vi "operate.vi"(8 "error in (no error)":errorcluster, 11 "reference in":refnum<class "GUI Controller.lvclass">) -> (0 "error out":errorcluster, 3 "reference out":refnum<class "GUI Controller.lvclass">)   [LabVIEW 2015, in "GUI Controller.lvclass"]
uses:
  GUI Controller.lvclass
  products.ctl
  inventory.ctl
  APP/excelFile_class/fileType.ctl
  followUp.ctl
  partsTracking.ctl
  state.ctl
  Project Panels_class/Project Panels.lvclass
  SYS/Items Controller_llb/Items Controller.lvclass
  APP/excelFile_class/excelFile.lvclass
  SYS/Notification Controller_class/Notification Controller.lvclass
  SYS/PartsTracking Controller_class/PartsTracking Controller.lvclass
  SYS/File Controller_llb/File Controller.lvclass
panel:
  out "Title":string
  in  "Parts Tracking":T1
  in  "Follow up":T2
  in  "fileType":T3
  in  "Settings Button":bool
  in  "Inventory":T4
  in  "Products":T5
  out "StatusBar":string
  in  "Stop Button":bool
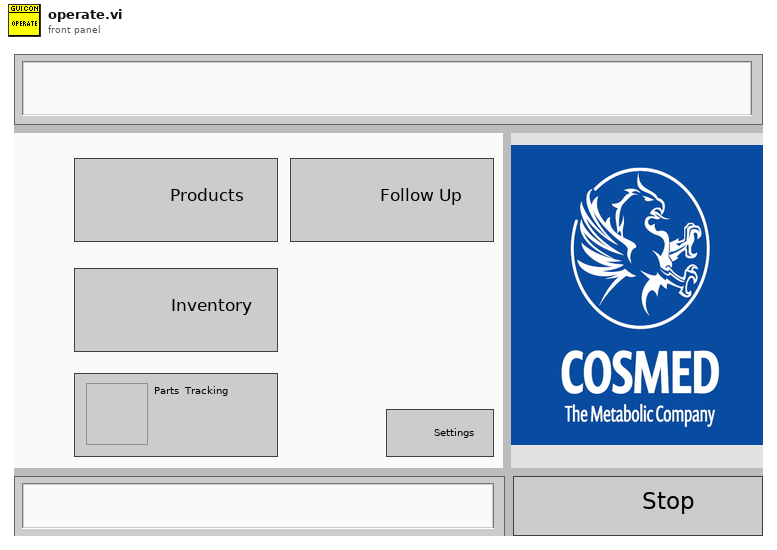
[diagram p1: front panel]
types:
  T1 = typedef "GUI Controller.lvclass/partsTracking.ctl" = bool
  T2 = typedef "GUI Controller.lvclass/followUp.ctl" = bool
  T3 = typedef "excelFile.lvclass/fileType.ctl" = enum16{"devices", "items", "partsTracking"}
  T4 = typedef "GUI Controller.lvclass/inventory.ctl" = bool
  T5 = typedef "GUI Controller.lvclass/products.ctl" = bool
  T6 = typedef "GUI Controller.lvclass/state.ctl" = enum16{"initiate", "checkNotificationItems", "checkNotificationTracking", "operate", "updateFromFile", "stop"}
  T7 = enum32{"Invalid", "Standard", "Closed", "Hidden", "Minimized", "Maximized"}
  T8 = typedef "GUI Controller.lvclass/ObjectAttributesRef.ctl" = refnum<data-value>
  T9 = typedef "GUI Controller.lvclass/ObjectAttributes.ctl" = cluster{"MyAttribute":dbl, "state":T6, "project_panels_ref":refnum<class "Project Panels.lvclass">, "items_controller_ref":refnum<class "Items Controller.lvclass">, "notification_controller_ref":refnum<class "Notification Controller.lvclass">, "partstracking_controller_ref":refnum<class "PartsTracking Controller.lvclass">, "file_controller_ref":refnum<class "File Controller.lvclass">}
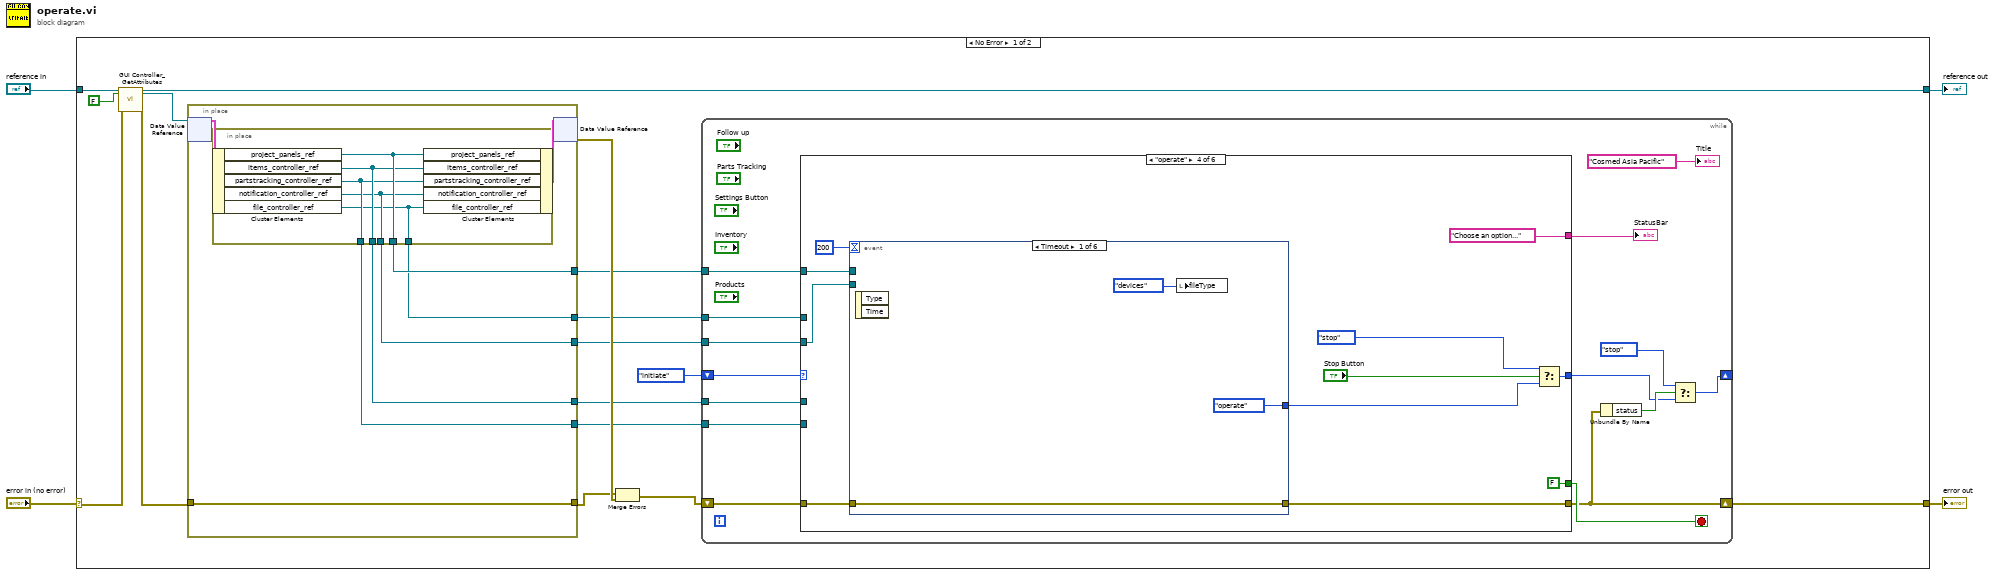
[diagram p0: block diagram]
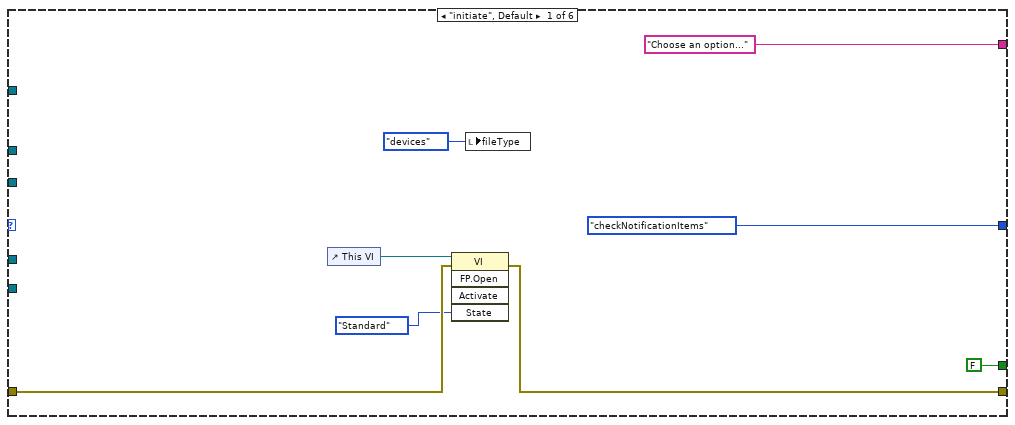
[diagram p2: hidden frame]
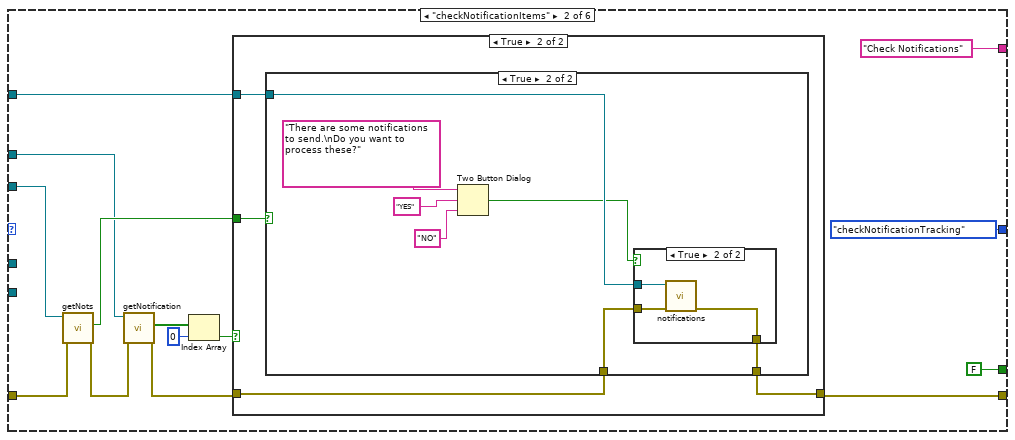
[diagram p3: hidden frame]
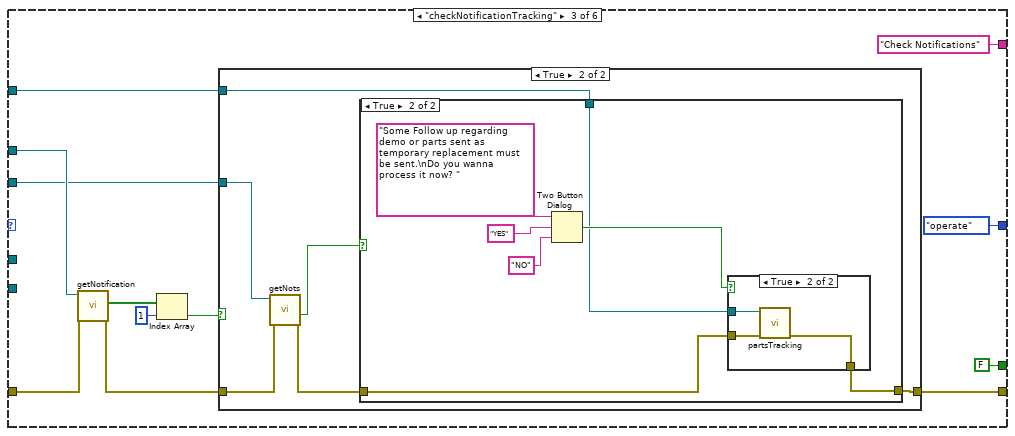
[diagram p7: hidden frame]
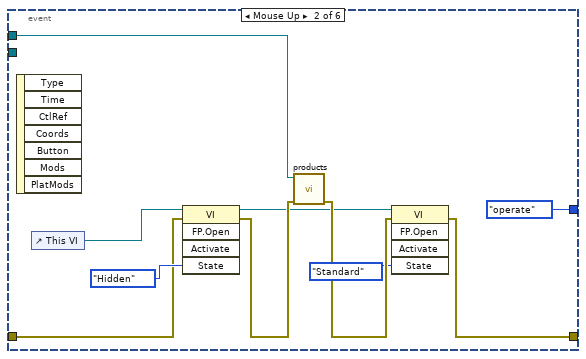
[diagram p11: hidden frame]
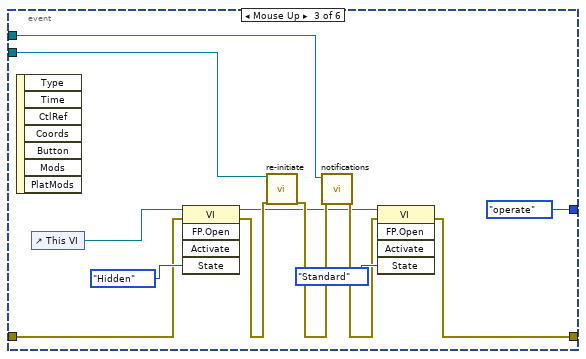
[diagram p12: hidden frame]
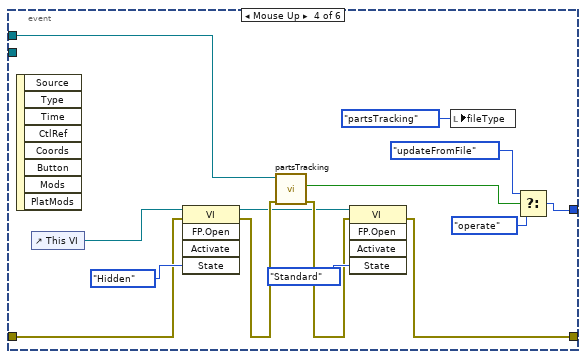
[diagram p13: hidden frame]
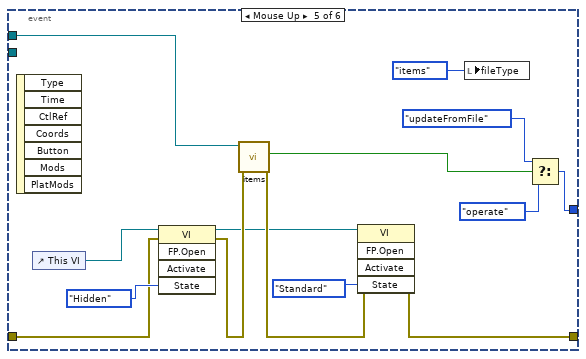
[diagram p14: hidden frame]
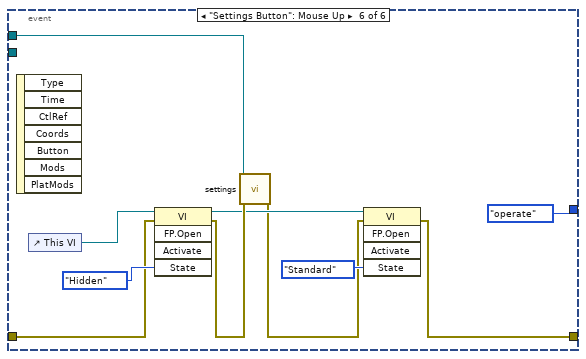
[diagram p15: hidden frame]
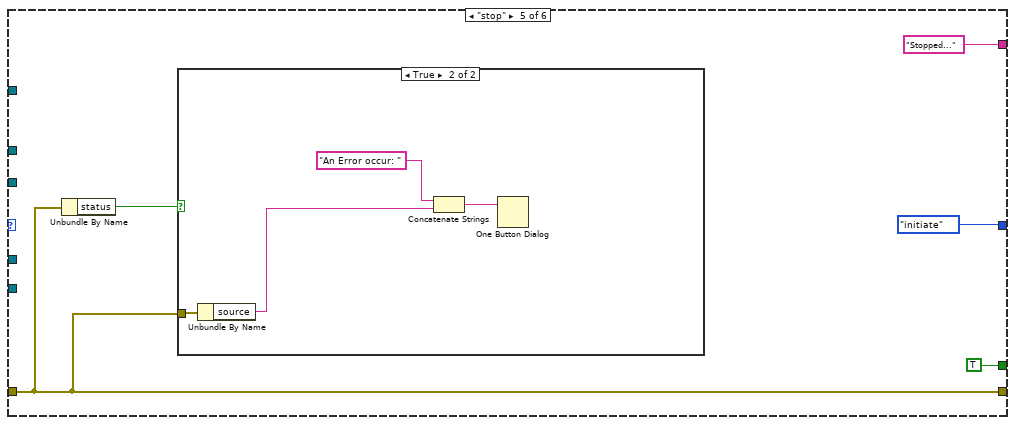
[diagram p16: hidden frame]
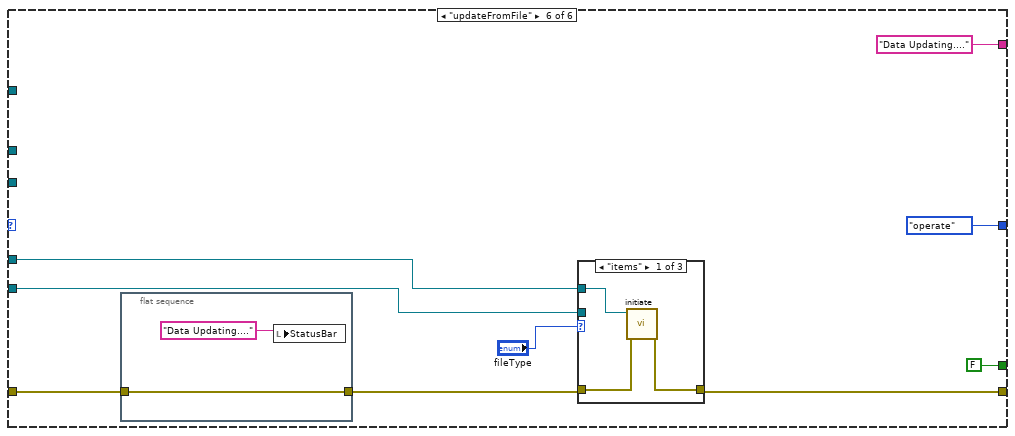
[diagram p18: hidden frame]
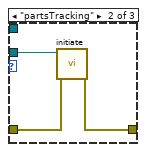
[diagram p19: hidden frame]
diagram:
  n1 = case shown="No Error" "error in (no error)" {
    selector: "error in (no error)" -> [w16 w221]
    tunnel: [w9 w221] -> w3
    tunnel: [w14 w220] -> w1
    tunnel: "reference in" -> [w18 w220]
    frame No Error {
      n2 = call "GUI Controller_GetAttributes.vi"("reference in"=w18, "return data? (T)"=FALSE, "error in (no error)"=w16) -> ("reference out"=w14:refnum<class "GUI Controller.lvclass">, "attributes ref"=w13:T8, "error out"=w15:errorcluster)  [unwired: 13 in, 1 out]
      n3 = in-place {
        in-place-border: w15 -> [w212]
        in-place-border: [w212] -> w19
        in-place-border: [w211] -> w10
        in-place-border: [w210] -> w8
        in-place-border: [w209] -> w7
        in-place-border: [w208] -> w6
        in-place-border: [w207] -> w5
        n4 = in-place-dvr #1(w13) -> (w213:T9)  [unwired: 1 out]
        n5 = in-place {
          in-place-border: [w219] -> w211
          in-place-border: [w218] -> w210
          in-place-border: [w217] -> w209
          in-place-border: [w216] -> w208
          in-place-border: [w215] -> w207
          n6 = in-place-cluster #2(w213) -> ("project_panels_ref"=w219:refnum<class "Project Panels.lvclass">, "items_controller_ref"=w218:refnum<class "Items Controller.lvclass">, "partstracking_controller_ref"=w217:refnum<class "PartsTracking Controller.lvclass">, "notification_controller_ref"=w216:refnum<class "Notification Controller.lvclass">, "file_controller_ref"=w215:refnum<class "File Controller.lvclass">)
          n7 = in-place-cluster #2("project_panels_ref"=w219, "items_controller_ref"=w218, "partstracking_controller_ref"=w217, "notification_controller_ref"=w216, "file_controller_ref"=w215) -> (w214:T9)
        }
        n8 = in-place-dvr #1(w214) -> (w20:errorcluster)  [unwired: 1 out]
      }
      n9 = Merge Errors(w19, w20) -> (w12:errorcluster)
      n10 = while {
        shift-right: [w28] -> _
        shift-left: state."initiate" ("state") -> [w34]
        shift-right: [w30] -> w9
        shift-left: w12 -> [w35]
        tunnel: w10 -> [w27]
        tunnel: w8 -> [w24]
        tunnel: w7 -> [w23]
        tunnel: w6 -> [w22]
        tunnel: w5 -> [w21]
        stop <- w31 stop-if-true
        n11 = case shown="\"operate\"" w34 {
          tunnel: w35 -> [w40 w54 w82 w111 w181 w190]
          tunnel: [w39 w51 w76 w110 w181 w194] -> w30
          tunnel: [state."checkNotificationItems" ("state") state."checkNotificationTracking" ("state") state."operate" ("state") w113 state."initiate" ("state") state."operate" ("state")] -> w26
          tunnel: ["Choose an option..." ("Title") "Check Notifications" ("Title") "Check Notifications" ("Title") "Choose an option..." ("Title") "Stopped..." ("Title") "Data Updating...." ("Title")] -> w33
          tunnel: [FALSE FALSE FALSE FALSE TRUE FALSE] -> w31
          tunnel: w27 -> [_ w52 w75 w108 _ _]
          tunnel: w24 -> [_ _ _ _ _ w192]
          tunnel: w23 -> [_ _ _ _ _ w191]
          tunnel: w22 -> [_ w55 w79 w106 _ _]
          tunnel: w21 -> [_ w49 w83 _ _ _]
          frame "initiate", Default {
            n12 = control-ref of="This VI"() -> (w41:refnum<vi>)
            n13 = invoke class="VI" method="FP.Open"(reference=w41, error in=w40, "State"=T7."Standard") -> (error out=w39:errorcluster)  [unwired: 2 in, 4 out]
            n14 = local write "fileType"(fileType."devices" ("fileType")) -> ()
          }
          frame "checkNotificationItems" {
            n15 = call "getNots.vi"("error in (no error)"=w54, "reference in"=w55) -> ("error out"=w48:errorcluster, "nots?"=w53:bool)  [unwired: 6 in, 2 out]
            n16 = call "getNotification.vi"("error in (no error)"=w48, "reference in"=w49) -> ("error out"=w47:errorcluster, "not_setting"=w46:bool[])  [unwired: 7 in, 1 out]
            n17 = Index Array(array=w46, index=0) -> (element=w45:bool)
            n18 = case shown="True" w45 {
              tunnel: w53 -> [_ w62]
              tunnel: w52 -> [_ w61]
              tunnel: [w58 w60] -> w51
              tunnel: w47 -> [w58 w59]
              frame False {
              }
              frame True {
                n19 = case shown="True" w62 {
                  tunnel: w61 -> [_ w67]
                  tunnel: w59 -> [w63 w66]
                  tunnel: [w63 w65] -> w60
                  frame False {
                  }
                  frame True {
                    n20 = Two Button Dialog(message="There are some notifications to send.\nDo you want to process these?", 1:"NO" ("F button name (\"Cancel\")"), 2:"YES" ("T button name (\"OK\")")) -> (T button?=w64:bool)
                    n21 = case shown="True" w64 {
                      tunnel: w67 -> [_ w74]
                      tunnel: w66 -> [w71 w73]
                      tunnel: [w71 w72] -> w65
                      frame False {
                      }
                      frame True {
                        n22 = call "notifications.vi"("error in (no error)"=w73, "reference in"=w74) -> ("error out"=w72:errorcluster)  [unwired: 7 in, 2 out]
                      }
                    }
                  }
                }
              }
            }
          }
          frame "checkNotificationTracking" {
            n23 = call "getNotification.vi"("error in (no error)"=w82, "reference in"=w83) -> ("error out"=w78:errorcluster, "not_setting"=w81:bool[])  [unwired: 7 in, 1 out]
            n24 = Index Array(array=w81, index=1) -> (element=w77:bool)
            n25 = case shown="True" w77 {
              tunnel: w79 -> [_ w93]
              tunnel: w78 -> [w87 w92]
              tunnel: [w87 w90] -> w76
              tunnel: w75 -> [_ w88]
              frame False {
              }
              frame True {
                n26 = call "getNots.vi"("error in (no error)"=w92, "reference in"=w93) -> ("error out"=w91:errorcluster, "tracking_nots?"=w89:bool)  [unwired: 6 in, 2 out]
                n27 = case shown="True" w89 {
                  tunnel: w91 -> [w94 w97]
                  tunnel: [w94 w96] -> w90
                  tunnel: w88 -> [_ w95]
                  frame False {
                  }
                  frame True {
                    n28 = Two Button Dialog(message="Some Follow up regarding demo or parts sent as temporary replacement must be sent.\nDo you wanna process it now? ", 1:"NO" ("F button name (\"Cancel\")"), 2:"YES" ("T button name (\"OK\")")) -> (T button?=w98:bool)
                    n29 = case shown="True" w98 {
                      tunnel: w97 -> [w102 w105]
                      tunnel: [w102 w104] -> w96
                      tunnel: w95 -> [_ w103]
                      frame False {
                      }
                      frame True {
                        n30 = call "partsTracking.vi"("error in (no error)"=w105, "reference in"=w103) -> ("error out"=w104:errorcluster)  [unwired: 7 in, 2 out]
                      }
                    }
                  }
                }
              }
            }
          }
          frame "operate" {
            n31 = event shown="[0] Timeout" {
              selector: _ -> [_ _ _ _ _ _]
              dyn-events: _ -> [_ _ _ _ _ _]
              timeout: 200 -> [_ _ _ _ _ _]
              tunnel: w111 -> [w117 w127 w139 w153 w167 w177]
              tunnel: [w117 w122 w131 w144 w157 w170] -> w110
              tunnel: w108 -> [_ w126 w138 w152 w166 w176]
              tunnel: [state."operate" ("f") state."operate" ("f") state."operate" ("f") w149 w161 state."operate" ("state")] -> w107
              tunnel: w106 -> [_ _ w134 _ _ _]
              event Timeout {
                n32 = event-data() -> ()  [unwired: 1 in, 2 out]
                n33 = local write "fileType"(fileType."devices" ("fileType")) -> ()
              }
              event Mouse Up {
                n34 = event-data() -> ()  [unwired: 1 in, 7 out]
                n35 = control-ref of="This VI"() -> (w129:refnum<vi>)
                n36 = invoke class="VI" method="FP.Open"(reference=w129, error in=w127, "State"=T7."Hidden") -> (reference out=w121:refnum<vi>, error out=w125:errorcluster)  [unwired: 2 in, 3 out]
                n37 = call "products.vi"("error in (no error)"=w125, "reference in"=w126) -> ("error out"=w123:errorcluster)  [unwired: 8 in, 1 out]
                n38 = invoke class="VI" method="FP.Open"(reference=w121, error in=w123, "State"=T7."Standard") -> (error out=w122:errorcluster)  [unwired: 2 in, 4 out]
              }
              event Mouse Up {
                n39 = event-data() -> ()  [unwired: 1 in, 7 out]
                n40 = control-ref of="This VI"() -> (w141:refnum<vi>)
                n41 = invoke class="VI" method="FP.Open"(reference=w141, error in=w139, "State"=T7."Hidden") -> (reference out=w130:refnum<vi>, error out=w136:errorcluster)  [unwired: 2 in, 3 out]
                n42 = call "re-initiate.vi"("reference in"=w134, "error in (no error)"=w136) -> ("error out"=w135:errorcluster)  [unwired: 16 in, 1 out]
                n43 = call "notifications.vi"("error in (no error)"=w135, "reference in"=w138) -> ("error out"=w132:errorcluster)  [unwired: 7 in, 2 out]
                n44 = invoke class="VI" method="FP.Open"(reference=w130, error in=w132, "State"=T7."Standard") -> (error out=w131:errorcluster)  [unwired: 2 in, 4 out]
              }
              event Mouse Up {
                n45 = event-data() -> ()  [unwired: 1 in, 8 out]
                n46 = control-ref of="This VI"() -> (w155:refnum<vi>)
                n47 = invoke class="VI" method="FP.Open"(reference=w155, error in=w153, "State"=T7."Hidden") -> (reference out=w142:refnum<vi>, error out=w151:errorcluster)  [unwired: 2 in, 3 out]
                n48 = call "partsTracking.vi"("error in (no error)"=w151, "reference in"=w152) -> ("error out"=w143:errorcluster, "saved?"=w150:bool)  [unwired: 7 in, 1 out]
                n49 = invoke class="VI" method="FP.Open"(reference=w142, error in=w143, "State"=T7."Standard") -> (error out=w144:errorcluster)  [unwired: 2 in, 4 out]
                n50 = local write "fileType"(fileType."partsTracking" ("fileType")) -> ()
                n51 = Select(t=state."updateFromFile" ("state"), s=w150, f=state."operate" ("state")) -> (s? t:f=w149:T6)
              }
              event Mouse Up {
                n52 = event-data() -> ()  [unwired: 1 in, 7 out]
                n53 = control-ref of="This VI"() -> (w168:refnum<vi>)
                n54 = invoke class="VI" method="FP.Open"(reference=w168, error in=w167, "State"=T7."Hidden") -> (reference out=w156:refnum<vi>, error out=w165:errorcluster)  [unwired: 2 in, 3 out]
                n55 = call "items.vi"("error in (no error)"=w165, "reference in"=w166) -> ("error out"=w158:errorcluster, "saved?"=w160:bool)  [unwired: 7 in, 1 out]
                n56 = invoke class="VI" method="FP.Open"(reference=w156, error in=w158, "State"=T7."Standard") -> (error out=w157:errorcluster)  [unwired: 2 in, 4 out]
                n57 = local write "fileType"(fileType."items" ("fileType")) -> ()
                n58 = Select(t=state."updateFromFile" ("state"), s=w160, f=state."operate" ("state")) -> (s? t:f=w161:T6)
              }
              event "Settings Button": Mouse Up {
                n59 = event-data() -> ()  [unwired: 1 in, 7 out]
                n60 = control-ref of="This VI"() -> (w178:refnum<vi>)
                n61 = invoke class="VI" method="FP.Open"(reference=w178, error in=w177, "State"=T7."Hidden") -> (reference out=w172:refnum<vi>, error out=w175:errorcluster)  [unwired: 2 in, 3 out]
                n62 = call "settings.vi"("error in (no error)"=w175, "reference in"=w176) -> ("error out"=w171:errorcluster)  [unwired: 8 in, 1 out]
                n63 = invoke class="VI" method="FP.Open"(reference=w172, error in=w171, "State"=T7."Standard") -> (error out=w170:errorcluster)  [unwired: 2 in, 4 out]
              }
            }
            n64 = Select(t=state."stop" ("state"), s="Stop Button", f=w107) -> (s? t:f=w113:T6)
          }
          frame "stop" {
            n65 = Unbundle By Name(w181) -> ("status"=w180:bool)
            n66 = case shown="True" w180 {
              tunnel: w181 -> [_ w186]
              frame False {
              }
              frame True {
                n67 = Unbundle By Name(w186) -> ("source"=w185:string)
                n68 = Concatenate Strings("An Error occur: " ("message"), w185) -> (w188:string)
                n69 = One Button Dialog(message=w188) -> ()  [unwired: 1 in, 1 out]
              }
            }
          }
          frame "updateFromFile" {
            n70 = flat-sequence {
              tunnel: w190 -> [w199]
              tunnel: [w199] -> w189
              frame #0 {
                n71 = local write "StatusBar"("Data Updating...." ("Title")) -> ()
              }
            }
            n72 = case shown="\"items\"" "fileType" {
              tunnel: w189 -> [w202 w205 w206]
              tunnel: [w201 w204 w206] -> w194
              tunnel: w192 -> [w200 _ _]
              tunnel: w191 -> [_ w203 _]
              frame "items" {
                n73 = call "initiate.vi"("error in (no error)"=w202, "reference in"=w200) -> ("error out"=w201:errorcluster)  [unwired: 8 in, 1 out]
              }
              frame "partsTracking" {
                n74 = call "initiate.vi"("error in (no error)"=w205, "reference in"=w203) -> ("error out"=w204:errorcluster)  [unwired: 8 in, 1 out]
              }
              frame "devices", Default {
              }
            }
          }
        }
        "StatusBar" <- w33
        n75 = Unbundle By Name(w30) -> ("status"=w29:bool)
        n76 = Select(t=state."stop", s=w29, f=w26) -> (s? t:f=w28:T6)
        "Title" <- "Cosmed Asia Pacific" ("Title")
      }
    }
    frame Error {
    }
  }
  "error out" <- w3
  "reference out" <- w1
